vi "Serial InitMarvin.vi"(8 "error in (no error)":errorcluster, 9 "VI reference (current VI)":refnum<vi>, 11 "VISA Refnum in":refnum<visa-resource-name>) -> (0 "error out":errorcluster, 3 "Boolean":bool)   [LabVIEW 2017]
uses:
  <vilib>/Instr/_visa.llb/VISA Configure Serial Port (Instr).vi
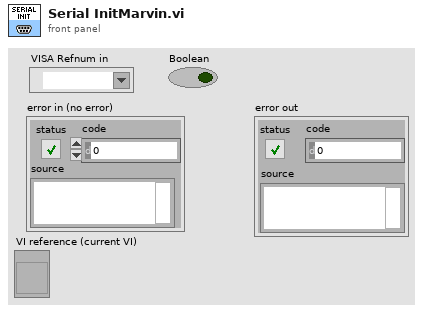
[diagram p1: front panel]
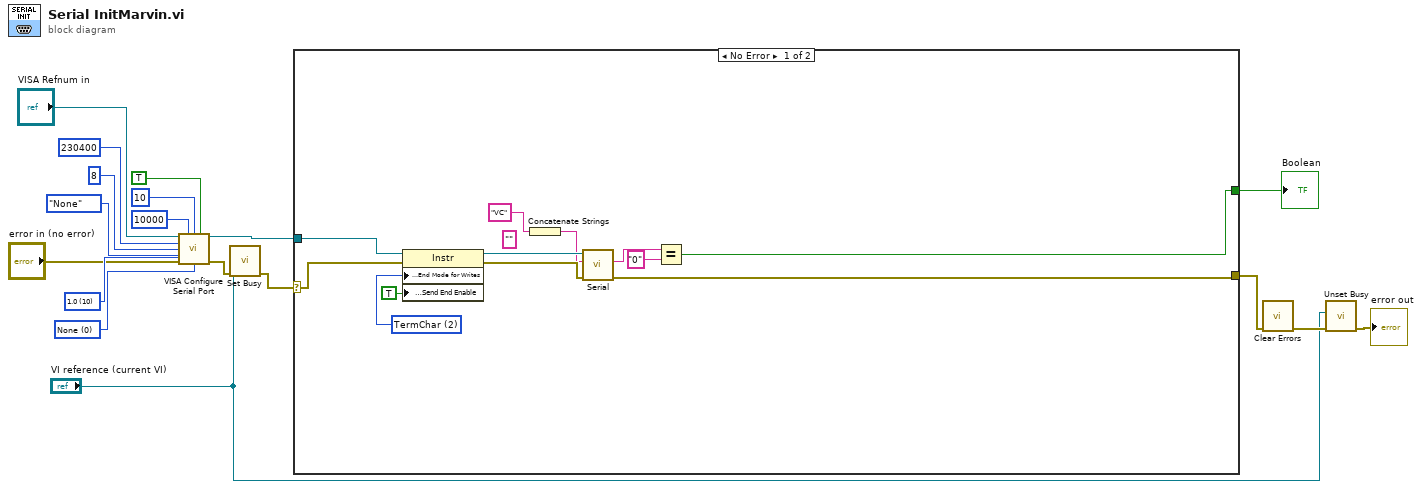
[diagram p0: block diagram]
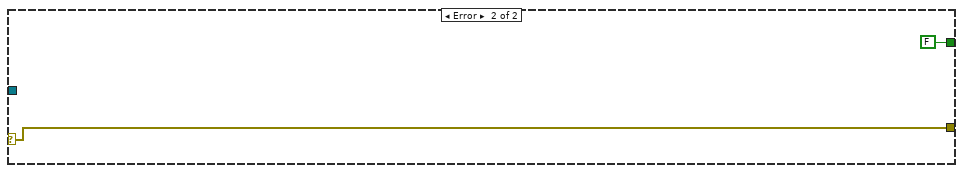
[diagram p2: hidden frame]
diagram:
  w15 = u16 0 items=["None", "XON/XOFF", "RTS/CTS", "XON/XOFF & RTS/CTS", "DTR/DSR", "XON/XOFF & DTR/DSR"] ("flow control (0:none)")
  w14 = u16 10 items=["1.0"=10, "1.5"=15, "2.0"=20] ("stop bits (10: 1 bit)")
  n1 = call-poly "VISA Configure Serial Port"("VISA resource name"="VISA Refnum in", "timeout (10sec)"=u32 10000, "termination char\n(0xA = '\\n' = LF)"=u8 10 ("termination char\n(0xA = '\\n' = LF)"), "Enable Termination\nChar (T)"=TRUE ("Enable Termination\nChar (T)"), "baud rate (9600)"=u32 230400, "data bits (8)"=u16 8, "parity (0:none)"=enum16{"None", "Odd", "Even", "Mark", "Space"}."None", "error in (no error)"="error in (no error)", "stop bits (10: 1 bit)"=w14, "flow control (0:none)"=w15) -> ("VISA resource name out"=w16:refnum<visa-resource-name>, "error out"=w5:errorcluster)  [unwired: 4 in]
  n2 = call <vilib>:"Set Busy.vi"("error in (no error)"=w5, "VI reference (current VI)"="VI reference (current VI)") -> ("error out"=w4:errorcluster)  [unwired: 8 in, 1 out]
  n3 = case shown="No Error" w4 {
    selector: w4 -> [w29 w31]
    tunnel: w16 -> [w30 _]
    tunnel: [w22 w31] -> w6
    tunnel: [w19 FALSE] -> w7
    frame No Error {
      (unwired) "" ("write buffer")
      w27 = u16 2 items=["None", "LastBit", "TermChar", "Break"] ("Serial Settings:Serial End Mode for Writes")
      n4 = property class="Instr"(reference=w30, error in=w29, "Serial Settings:End Mode for Writes"=w27, "Message Based Settings:Send End Enable"=TRUE) -> (reference out=w25:refnum<visa-resource-name>, error out=w26:errorcluster)
      n5 = Concatenate Strings("VC" ("string")) -> (w23:string)
      n6 = call "Serial.vi"("error in (no error)"=w26, "write buffer"=w23, "VISA resource name"=w25) -> ("error out"=w22:errorcluster, "read buffer"=w21:string)  [unwired: 7 in]
      n7 = Equal?(x=w21, y="0") -> (x = y?=w19:bool)
    }
    frame Error {
    }
  }
  "Boolean" <- w7
  n8 = call <vilib>:"Clear Errors.vi"("error in (no error)"=w6) -> ("error out"=w3:errorcluster)  [unwired: 5 in, 1 out]
  n9 = call <vilib>:"Unset Busy.vi"("error in (no error)"=w3, "VI reference (current VI)"="VI reference (current VI)") -> ("error out"=→"error out":errorcluster)  [unwired: 9 in]
